vi "Send Command.vi"(8 "error in (no error)":errorcluster, 9 "Value":string, 10 "Message":string, 11 "VISA resource name":refnum<visa-resource-name>) -> (0 "error out":errorcluster, 3 "VISA resource out":refnum<visa-resource-name>)   [LabVIEW 2011, in "Ocean Server OS4000.lvlib"]
doc: "Sends Command to the Instrument.\n<b> Message </b> is the command to be sent to the instrument.\n<b> Value </b> is the number to be sent to the instrument along with the command."
uses:
  Ocean Server OS4000.lvlib
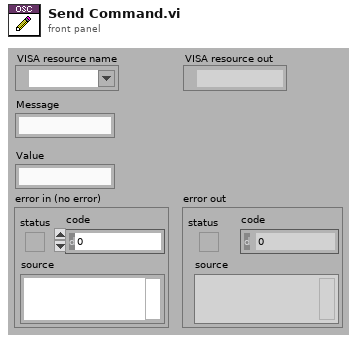
[diagram p1: front panel]
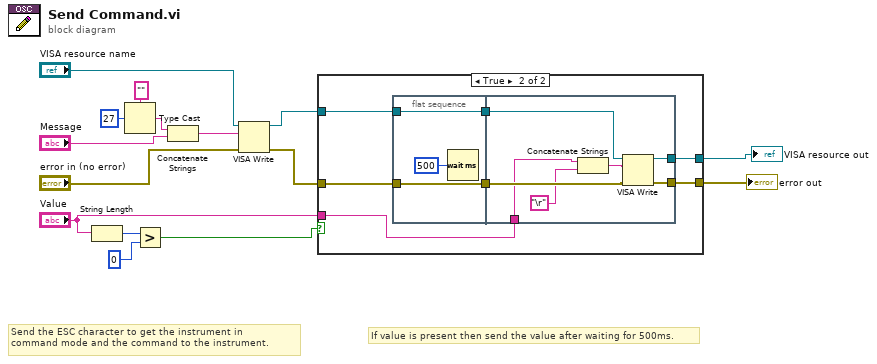
[diagram p0: block diagram]
diagram:
  # "If value is present then send the value after waiting for 500ms."
  # "Send the ESC character to get the instrument in\ncommand mode and the command to the instrument."
  n1 = String Length(string="Value") -> (length=w13:i32)
  n2 = Type Cast(type="", x=u8 27) -> (*(type *) &x=w4:string)
  n3 = Greater?(x=w13, y=0) -> (0:w11:bool)
  n4 = Concatenate Strings(w4, "Message") -> (w3:string)
  n5 = VISA Write(VISA resource name="VISA resource name", write buffer=w3, error in (no error)="error in (no error)") -> (VISA resource name out=w1:refnum<visa-resource-name>, error out=w2:errorcluster)  [unwired: 1 out]
  n6 = case shown="True" w11 {
    tunnel: w1 -> [w17 w24]
    tunnel: [w17 w23] -> w10
    tunnel: w2 -> [w16 w22]
    tunnel: [w16 w21] -> w8
    tunnel: "Value" -> [_ w18]
    frame False {
    }
    frame True {
      n7 = flat-sequence {
        tunnel: w22 -> [w26]
        tunnel: w24 -> [w27]
        tunnel: [w27] -> w20
        tunnel: [w26] -> w19
        tunnel: [w32] -> w23
        tunnel: [w30] -> w21
        tunnel: w20 -> [w33]
        tunnel: w19 -> [w31]
        tunnel: w18 -> [w28]
        frame #0 {
          n8 = Wait (ms)(milliseconds to wait=u32 500) -> ()  [unwired: 1 out]
        }
        frame #1 {
          n9 = Concatenate Strings(w28, "\r" ("Carriage Return Constant")) -> (w34:string)
          n10 = VISA Write(VISA resource name=w33, write buffer=w34, error in (no error)=w31) -> (VISA resource name out=w32:refnum<visa-resource-name>, error out=w30:errorcluster)  [unwired: 1 out]
        }
      }
    }
  }
  "VISA resource out" <- w10
  "error out" <- w8
